vi "StringLen.vi"(4 "String":refnum<class "Abs_String.lvclass">) -> (1 "Result":refnum<class "Abs_I32 Integer.lvclass">)   [LabVIEW 2021]
uses:
  Abs_Types/String/Abs_String.lvclass
  Abs_Types/I32 Integer/Abs_I32 Integer.lvclass
  Support/StringLen/StringLen_I32.lvclass
  C:/Program Files (x86)/National Instruments/LabVIEW 2021/vi.lib/TSA/Abstract Data Classes/Abs_Types/I32 Integer/Abs_I32 Integer.lvclass
  Support/StringLen/StringLen_I32.lvclass/StringLen_I32.ctl
  Support/StringLen/Properties/Write String.vi
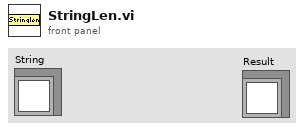
[diagram p1: front panel]
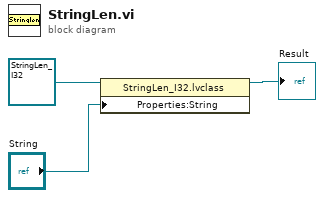
[diagram p0: block diagram]
diagram:
  n1 = property class="StringLen_I32.lvclass"(reference=refnum<class "StringLen_I32.lvclass"> refnum ("StringLen_I32.lvclass"), "Properties:String"="String") -> (reference out=→"Result":refnum<class "StringLen_I32.lvclass">)  [unwired: 1 in, 1 out]
